vi "SelectBackground.vi"() -> ()   [LabVIEW 2014]
uses:
  <vilib>/vision/driver/NI_Vision_Acquisition_Software.lvlib
panel:
  in  "base path":path=path "C:/Users/nagellab/Documents/LabView"
  in  "Select Bkd?":bool
  out "Background":T1(plugin-control)
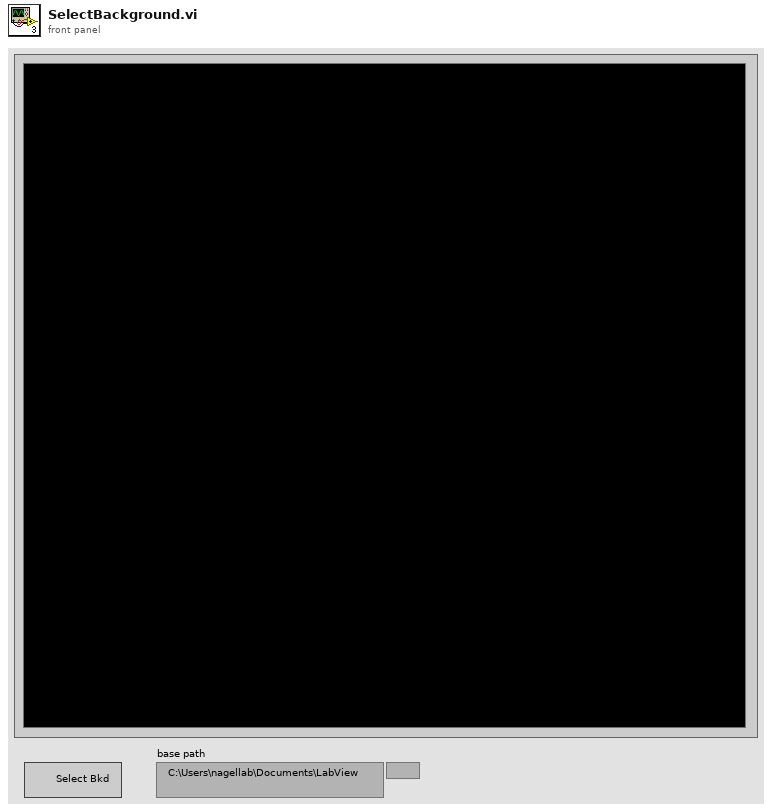
[diagram p1: front panel]
types:
  T1 = typedef "IMAQ Image.ctl" = refnum<image>
  T2 = typedef "IMAQdx.ctl" = refnum<k21>
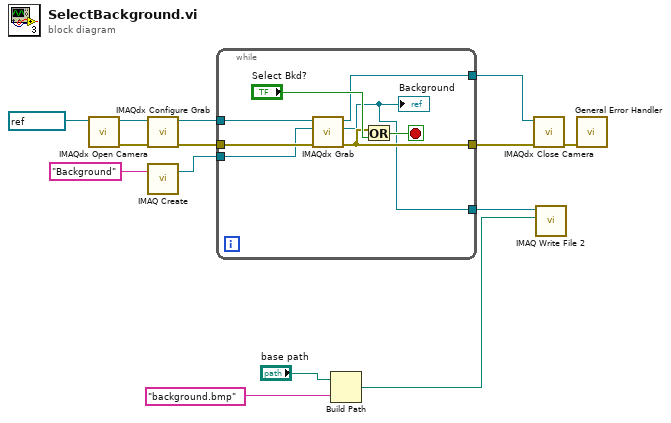
[diagram p0: block diagram]
diagram:
  n1 = call <vilib>:"IMAQdx Open Camera.vi"("Session In"=refnum<k21> "cam8" ("Camera Name")) -> ("error out"=w1:errorcluster, "Session Out"=w2:T2)  [unwired: 2 in, 7 out]
  n2 = call <vilib>:"IMAQdx Configure Grab.vi"("error in"=w1, "Session In"=w2) -> ("error out"=w12:errorcluster, "Session Out"=w13:T2)  [unwired: 8 out]
  n3 = call "IMAQ Create"("Image Name"="Background") -> ("New Image"=w14:T1)  [unwired: 3 in, 2 out]
  n4 = while {
    tunnel: [w17] -> w11
    tunnel: w12 -> [w19]
    tunnel: w13 -> [w20]
    tunnel: [w16] -> w10
    tunnel: w14 -> [w18]
    tunnel: [w15] -> w6
    stop <- w22 stop-if-true
    n5 = call <vilib>:"IMAQdx Grab.vi"("error in"=w19, "Image In"=w18, "Session In"=w20) -> ("error out"=w16:errorcluster, "Image Out"=w15:T1, "Session Out"=w17:T2)  [unwired: 1 in, 5 out]
    "Background" <- w15
    n6 = Or(x=w16, y="Select Bkd?") -> (x .or. y?=w22:bool)
  }
  n7 = Build Path(base path="base path", name or relative path="background.bmp" ("element")) -> (appended path=w4:path)
  n8 = call <vilib>:"IMAQdx Close Camera.vi"("error in"=w10, "Session In"=w11) -> ("error out"=w7:errorcluster)  [unwired: 9 out]
  n9 = call-poly "IMAQ Write File 2"("File Path"=w4, "Image"=w6) -> ()  [unwired: 8 in, 2 out]
  n10 = call <vilib>:"General Error Handler.vi"("error in (no error)"=w7) -> ()  [unwired: 2 in, 13 out]
